vi "Parse Messages.vi"(11 "Body":string) -> (3 "Messages":T1[](array[typedef]))   [LabVIEW 2015, in "NI_Azure_Queue.lvlib"]
uses:
  NI_Azure_Queue.lvlib
  Message.ctl
  XML Parsing/NI_Azure_XML Parsing.lvlib
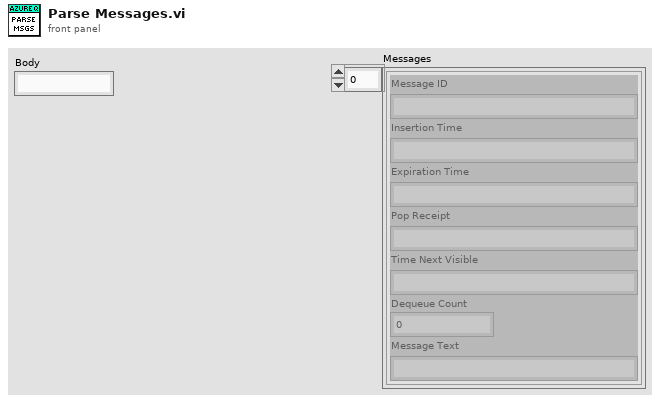
[diagram p1: front panel]
types:
  T1 = typedef "NI_Azure_Queue.lvlib/Message.ctl" = cluster{"Message ID":string, "Insertion Time":string, "Expiration Time":string, "Pop Receipt":string, "Time Next Visible":string, "Dequeue Count":i32, "Message Text":string}
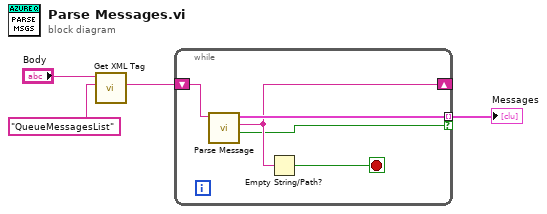
[diagram p0: block diagram]
diagram:
  n1 = call "Get XML Tag.vi"("Tag name"="QueueMessagesList", "XML String in"="Body") -> ("Tag value"=w2:string)  [unwired: 5 in, 4 out]
  n2 = while {
    tunnel: [w8] -> w1 mode=indexing if=w5
    shift-right: [w6] -> _
    shift-left: w2 -> [w9]
    stop <- w7 stop-if-true
    n3 = call "Parse Message.vi"("Body"=w9) -> ("found?"=w5:bool, "Remaining string"=w6:string, "Message"=w8:T1)  [unwired: 8 in]
    n4 = Empty String/Path?(string/path=w6) -> (empty?=w7:bool)
  }
  "Messages" <- w1
